vi "Open Help PDF.vi"(8 "error in":errorcluster, 10 "NewVal":bool, 11 "Path after documentation":path) -> (0 "error out":errorcluster)   [LabVIEW 2025, in "CAN-LIN Raw Bus Capture UI.lvlib"]
doc: "Opens the Help PDF in the designated sub-path of the installed documentation library."
uses:
  CAN-LIN Raw Bus Capture UI.lvlib
  <vilib>/Utility/sysdir.llb/System Directory Type.ctl
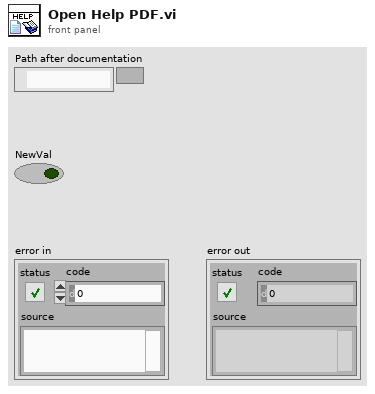
[diagram p1: front panel]
types:
  T1 = typedef "System Directory Type.ctl" = i32
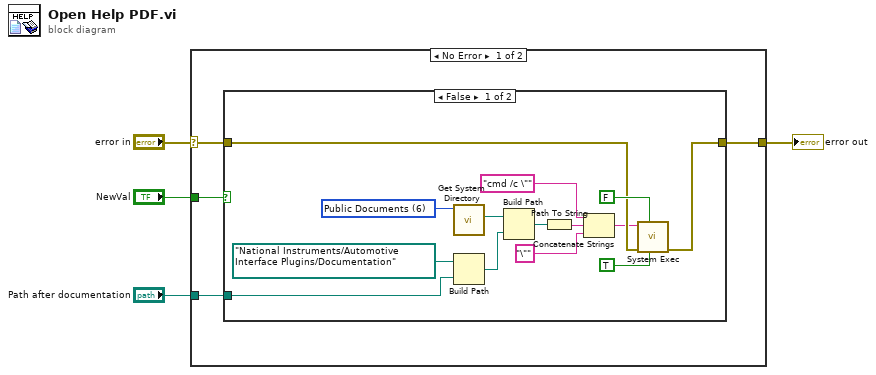
[diagram p0: block diagram]
diagram:
  n1 = case shown="No Error" "error in" {
    selector: "error in" -> [w6 w24]
    tunnel: "Path after documentation" -> [w8 _]
    tunnel: "NewVal" -> [w7 _]
    tunnel: [w5 w24] -> w4
    frame No Error {
      n2 = case shown="False" w7 {
        tunnel: [w12 w23] -> w5
        tunnel: w6 -> [w14 w23]
        tunnel: w8 -> [w9 _]
        frame False {
          w22 = T1 6 items=["User Home"=0, "User Desktop"=1, "User Documents"=2, "User Application Data"=3, "User Preferences"=4, "User Temporary"=5, "Public Documents"=6, "Public Application Data"=7, "Public Preferences"=8, "Public Cache"=13, "System Core Libraries"=9, "System Installed Libraries"=10, "Application Files"=11, "Boot Volume Root"=12] ("system directory type")
          n3 = call <vilib>:"Get System Directory.vi"("system directory type"=w22) -> ("system directory"=w21:path)  [unwired: 10 in]
          n4 = Build Path(base path=path "National Instruments/Automotive Interface Plugins/Documentation", name or relative path=w9) -> (appended path=w11:path)
          n5 = Build Path(base path=w21, name or relative path=w11) -> (appended path=w20:path)
          n6 = Path To String(path=w20) -> (string=w18:string)
          n7 = Concatenate Strings("cmd /c \"", w18, "\"") -> (w13:string)
          n8 = call <vilib>:"System Exec.vi"("run minimized? (F)"=TRUE, "wait until completion? (T)"=FALSE, "error in (no error)"=w14, "command line"=w13) -> ("error out"=w12:errorcluster)  [unwired: 4 in, 3 out]
        }
        frame True {
        }
      }
    }
    frame Error {
    }
  }
  "error out" <- w4
